vi "GetPackets.vi"(11 "ContextIn":T1={"COMHandler"="", "COMConfig"={"BaudRate"=9600, "DataBits"=8, "Parity"=enum."None", "StopBits"=10, "DataTransferTimeout[ms]"=10000, "FastTransferTimeout[ms]"=100, "Retries"=0, "MsWaitBeforeRetry"=0}, "HelloResponse"="", "DeviceDetected"=FALSE, "TransferRefusedByUser"=FALSE, "MeasurementFrequency"=0, "AvailablePacketsNr"=0, "RequestType"=enum."NONE", "Response"="", "DownloadSuccess"=FALSE, "PacketNames"=[], "Packets"=[], "ActivePacketID"=0} {"COMConfig"."StopBits" items=["1.0"=10, "1.5"=15, "2.0"=20]; "COMConfig"."DataBits" min=7 max=9 step=1; "COMConfig"."BaudRate" min=9600 max=921600 step=1}) -> (3 "ContextOut":T1={"COMHandler"="", "COMConfig"={"BaudRate"=9600, "DataBits"=8, "Parity"=enum."None", "StopBits"=10, "DataTransferTimeout[ms]"=10000, "FastTransferTimeout[ms]"=100, "Retries"=0, "MsWaitBeforeRetry"=0}, "HelloResponse"="", "DeviceDetected"=FALSE, "TransferRefusedByUser"=FALSE, "MeasurementFrequency"=0, "AvailablePacketsNr"=0, "RequestType"=enum."NONE", "Response"="", "DownloadSuccess"=FALSE, "PacketNames"=[], "Packets"=[], "ActivePacketID"=0} {"COMConfig"."StopBits" items=["1.0"=10, "1.5"=15, "2.0"=20]; "COMConfig"."DataBits" min=7 max=9 step=1; "COMConfig"."BaudRate" min=9600 max=921600 step=1})   [LabVIEW 2016]
doc: "Get all available packets. Packet by packet, decoding data frame on the fly."
uses:
  FSContext.ctl
  FTDI/COMConfig.ctl
  Requests/RequestType.ctl
  Packet.ctl
  Sample.ctl
  Reading.ctl
  ReadingUnits/AccelReadingUnit.ctl
  ReadingUnits/GyroReadingUnit.ctl
  GetPackets/GPState.ctl
  GetPackets/GPContext.ctl
panel:
  out "seconds remaining":u32
  out "Prompt":string
  in  "Download failed!":bool
  out "DownloadStatus":u8(slide) scale=0.0..99.0
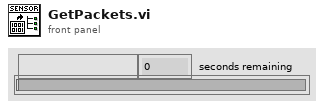
[diagram p1: front panel]
types:
  T1 = typedef "FSContext.ctl" = cluster{"COMHandler":refnum<visa-resource-name>, "COMConfig":T2, "HelloResponse":string, "DeviceDetected":bool, "TransferRefusedByUser":bool, "MeasurementFrequency":u32, "AvailablePacketsNr":u32, "RequestType":T3, "Response":string, "DownloadSuccess":bool, "PacketNames":string[], "Packets":T4[], "ActivePacketID":i32}
  T2 = typedef "COMConfig.ctl" = cluster{"BaudRate":u32, "DataBits":u16, "Parity":enum16{"None", "Odd", "Even", "Mark", "Space"}, "StopBits":u16, "DataTransferTimeout[ms]":u32, "FastTransferTimeout[ms]":u32, "Retries":i32, "MsWaitBeforeRetry":u32}
  T3 = typedef "RequestType.ctl" = enum16{"NONE", "Reset", "Hello", "GetPacketsNr", "GetMeasFreq", "GetPacket", "Goodbye"}
  T4 = typedef "Packet.ctl" = cluster{"Name":string, "SamplesNr":u32, "Samples":T5[], "AccelReadingUnit":T7, "GyroReadingUnit":T8}
  T5 = typedef "Sample.ctl" = cluster{"Accel":T6, "Gyro":T6}
  T6 = typedef "Reading.ctl" = cluster{"X":dbl, "Y":dbl, "Z":dbl}
  T7 = typedef "AccelReadingUnit.ctl" = enum16{"INVALID", "RAW", "g"}
  T8 = typedef "GyroReadingUnit.ctl" = enum16{"INVALID", "RAW", "°/sec"}
  T9 = typedef "GPContext.ctl" = cluster{"PacketsDownloaded":u32, "Millisecond":u32, "PacketsAfterNextSecond":u32}
  T10 = typedef "GPState.ctl" = enum16{"IDLE", "HandleErrors", "Init", "GetPacket", "UpdateDownloadSpeed", "UpdateProgress", "Stop"}
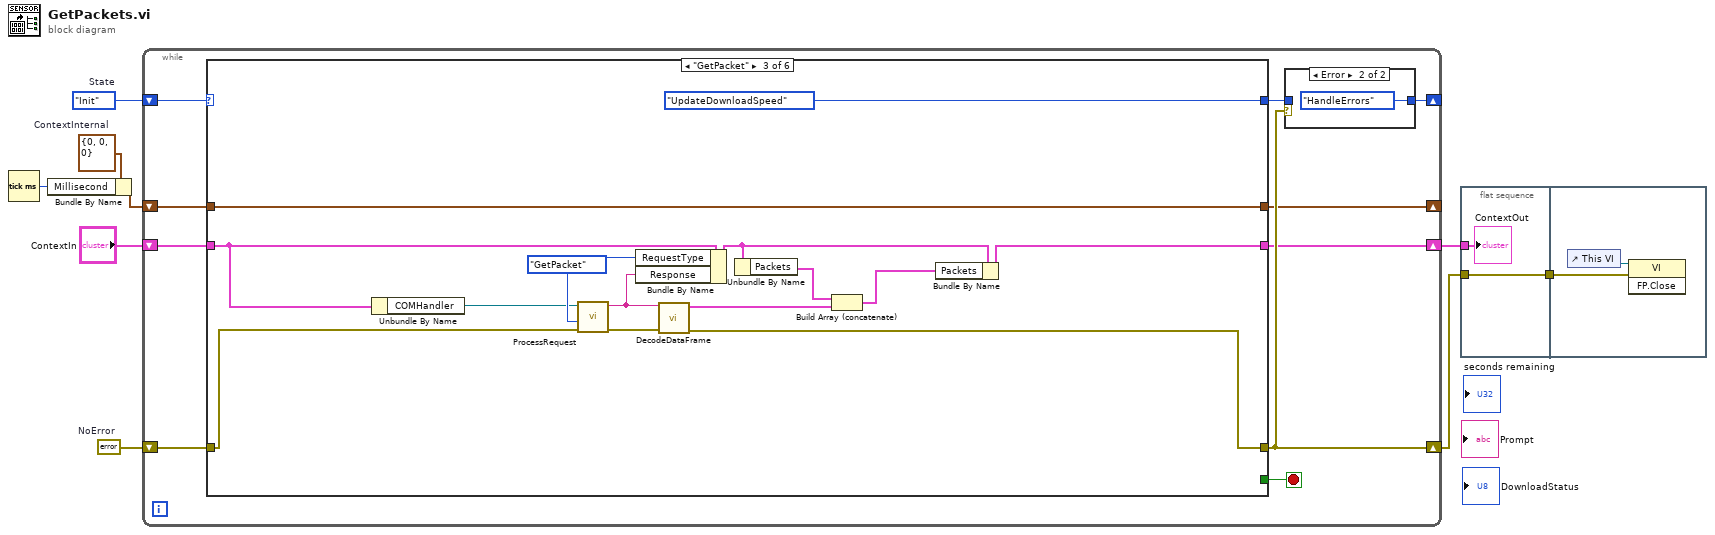
[diagram p0: block diagram]
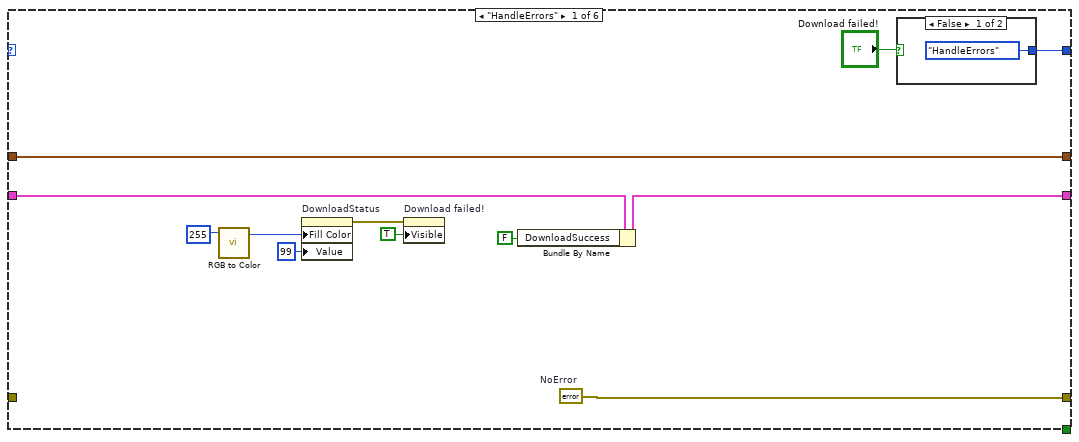
[diagram p3: hidden frame]
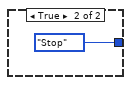
[diagram p4: hidden frame]
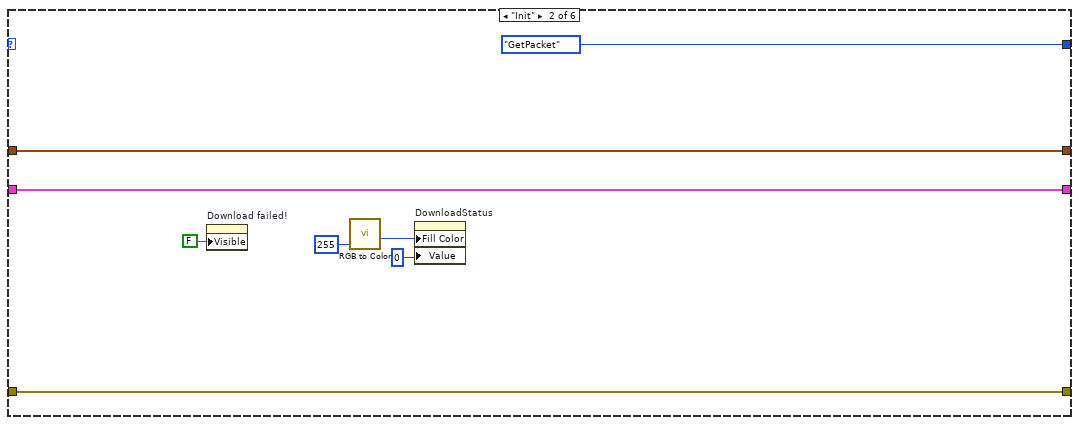
[diagram p5: hidden frame]
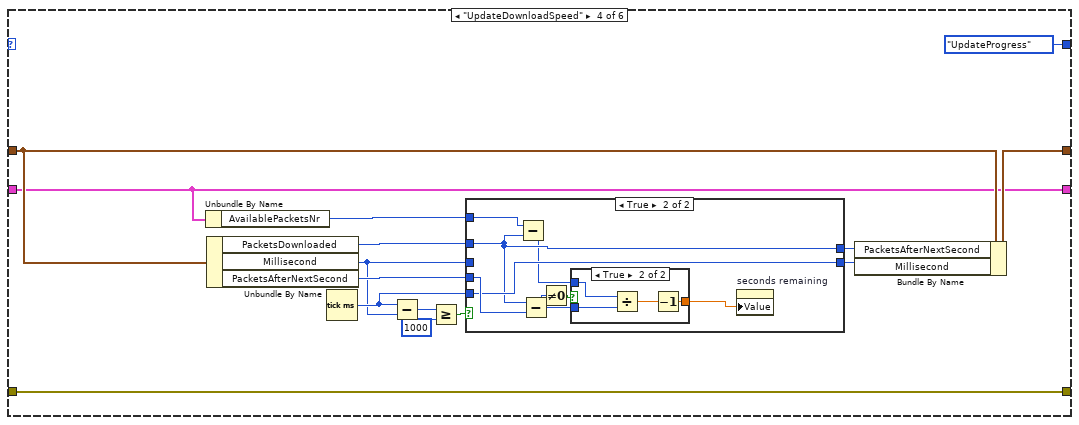
[diagram p6: hidden frame]
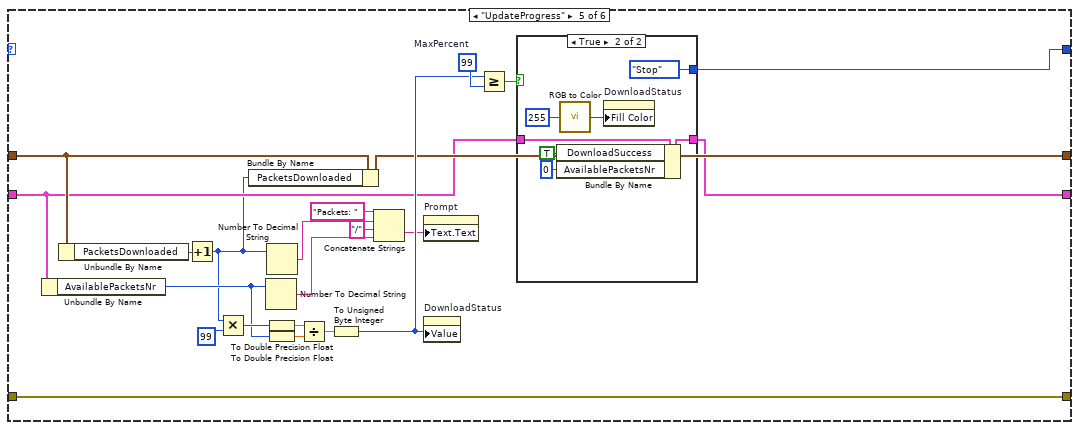
[diagram p9: hidden frame]
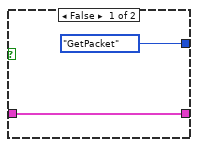
[diagram p10: hidden frame]
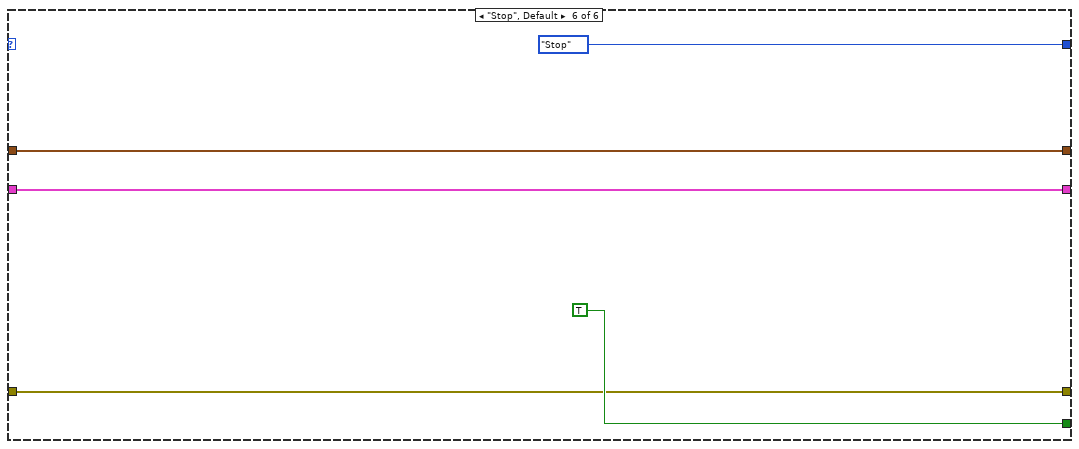
[diagram p11: hidden frame]
diagram:
  w4 = T9 {"PacketsDownloaded"=0, "Millisecond"=0, "PacketsAfterNextSecond"=0}  # ContextInternal
  w8 = errorcluster {"status"=FALSE, "code"=0, "source"=""}  # NoError
  w1 = GPState."Init"  # State
  n1 = Tick Count (ms)() -> (millisecond timer value=w3:u32)
  n2 = Bundle By Name(cluster=w4, "Millisecond"=w3) -> (w2:T9)
  n3 = while {
    shift-right: [w10] -> _
    shift-left: w1 -> [w11]
    shift-right: [w12] -> w7
    shift-left: "ContextIn" -> [w19]
    shift-right: [w15] -> w6
    shift-left: w8 -> [w18]
    shift-right: [w13] -> _
    shift-left: w2 -> [w14]
    stop <- w16 stop-if-true
    n4 = case shown="\"GetPacket\"" w11 {
      tunnel: w19 -> [w23 w41 w54 w59 w89 w120]
      tunnel: w18 -> [_ w43 w55 w62 w99 w121]
      tunnel: [w25 w43 w44 w62 w99 w121] -> w15
      tunnel: [w33 GPState."GetPacket" ("State") GPState."UpdateDownloadSpeed" ("State") GPState."UpdateProgress" ("State") w100 GPState."Stop" ("State")] -> w17
      tunnel: [_ _ _ _ _ TRUE] -> w16
      tunnel: [w22 w41 w45 w59 w88 w120] -> w12
      tunnel: w14 -> [w32 w36 w52 w65 w91 w118]
      tunnel: [w32 w36 w52 w64 w90 w118] -> w13
      frame "HandleErrors" {
        w25 = errorcluster {"status"=FALSE, "code"=0, "source"=""}  # NoError
        n5 = call <vilib>:"RGB to Color.vi"("R"=u8 255 ("G")) -> ("Color"=w30:u32)  [unwired: 2 in]
        n6 = property on="DownloadStatus" class="Slide (strict)"("Fill Color"=w30, "Value"=u8 99 ("DownloadStatus")) -> (error out=w29:errorcluster)  [unwired: 2 in, 1 out]
        n7 = property on="Download failed!" class="Bool"(error in=w29, "Visible"=TRUE) -> ()  [unwired: 1 in, 2 out]
        n8 = Bundle By Name(cluster=w23, "DownloadSuccess"=FALSE) -> (w22:T1)
        n9 = case shown="False" "Download failed!" {
          tunnel: [GPState."HandleErrors" ("State") GPState."Stop" ("State")] -> w33
          frame False {
          }
          frame True {
          }
        }
      }
      frame "Init" {
        n10 = property on="Download failed!" class="Bool"("Visible"=FALSE) -> ()  [unwired: 2 in, 2 out]
        n11 = call <vilib>:"RGB to Color.vi"("B"=u8 255 ("G")) -> ("Color"=w39:u32)  [unwired: 2 in]
        n12 = property on="DownloadStatus" class="Slide (strict)"("Fill Color"=w39, "Value"=u8 0 ("DownloadStatus")) -> ()  [unwired: 2 in, 2 out]
      }
      frame "GetPacket" {
        w57 = RequestType."GetPacket" ("RequestType")
        n13 = Unbundle By Name(w54) -> ("COMHandler"=w56:refnum<visa-resource-name>)
        n14 = call "ProcessRequest.vi"("ErrorIn"=w55, "RequestType"=w57, "DeviceResourceName"=w56) -> ("ErrorOut"=w50:errorcluster, "Response"=w51:string)  [unwired: 5 in, 2 out]
        n15 = Bundle By Name(cluster=w54, "RequestType"=w57, "Response"=w51) -> (w46:T1)
        n16 = call "DecodeDataFrame.vi"("ErrorIn"=w50, "Frame"=w51) -> ("ErrorOut"=w44:errorcluster, "Packets"=w49:T4[])  [unwired: 8 in]
        n17 = Unbundle By Name(w46) -> ("Packets"=w48:T4[])
        n18 = Build Array (concatenate)(w48, w49) -> (w47:T4[])
        n19 = Bundle By Name(cluster=w46, "Packets"=w47) -> (w45:T1)
      }
      frame "UpdateDownloadSpeed" {
        n20 = Unbundle By Name(w59) -> ("AvailablePacketsNr"=w58:u32)
        n21 = Unbundle By Name(w65) -> ("PacketsDownloaded"=w68:u32, "Millisecond"=w60:u32, "PacketsAfterNextSecond"=w69:u32)
        n22 = Tick Count (ms)() -> (millisecond timer value=w61:u32)
        n23 = Subtract(x=w61, y=w60) -> (x-y=w72:u32)
        n24 = Greater Or Equal?(x=w72, y=u32 1000) -> (x >= y?=w70:bool)
        n25 = case shown="True" w70 {
          tunnel: w69 -> [w73 w82]
          tunnel: w68 -> [_ w79]
          tunnel: [w73 w79] -> w67
          tunnel: w60 -> [w74 _]
          tunnel: [w74 w81] -> w66
          tunnel: w61 -> [_ w81]
          tunnel: w58 -> [_ w80]
          frame False {
          }
          frame True {
            n26 = Subtract(x=w80, y=w79) -> (x-y=w76:u32)
            n27 = Subtract(x=w79, y=w82) -> (x-y=w77:u32)
            n28 = Not Equal To 0?(x=w77) -> (x != 0?=w78:bool)
            n29 = case shown="True" w78 {
              tunnel: w77 -> [_ w85]
              tunnel: w76 -> [_ w86]
              tunnel: [_ w83] -> w75
              frame False {
              }
              frame True {
                n30 = Divide(x=w86, y=w85) -> (x/y=w84:dbl)
                n31 = Decrement(x=w84) -> (x-1=w83:dbl)
              }
            }
            n32 = property on="seconds remaining" class="DigNum (strict)"("Value"=w75) -> ()  [unwired: 2 in, 2 out]
          }
        }
        n33 = Bundle By Name(cluster=w65, "PacketsAfterNextSecond"=w67, "Millisecond"=w66) -> (w64:T9)
      }
      frame "UpdateProgress" {
        w103 = u8 99  # MaxPercent
        n34 = Unbundle By Name(w89) -> ("AvailablePacketsNr"=w93:u32)
        n35 = Unbundle By Name(w91) -> ("PacketsDownloaded"=w92:u32)
        n36 = Increment(x=w92) -> (x+1=w87:u32)
        n37 = Multiply(x=w87, y=u32 99) -> (x*y=w107:u32)
        n38 = Bundle By Name(cluster=w91, "PacketsDownloaded"=w87) -> (w90:T9)
        n39 = Number To Decimal String(number=w93) -> (decimal integer string=w97:string)  [unwired: 1 in]
        n40 = Number To Decimal String(number=w87) -> (decimal integer string=w96:string)  [unwired: 1 in]
        n41 = To Double Precision Float(number=w107) -> (double precision float=w106:dbl)
        n42 = To Double Precision Float(number=w93) -> (double precision float=w105:dbl)
        n43 = Divide(x=w106, y=w105) -> (x/y=w104:dbl)
        n44 = To Unsigned Byte Integer(number=w104) -> (unsigned 8bit integer=w102:u8)
        n45 = Concatenate Strings("Packets: " ("string"), w96, "/" ("string"), w97) -> (w98:string)
        n46 = property on="Prompt" class="Str"("Text.Text"=w98) -> ()  [unwired: 2 in, 2 out]
        n47 = property on="DownloadStatus" class="Slide (strict)"("Value"=w102) -> ()  [unwired: 2 in, 2 out]
        n48 = Greater Or Equal?(x=w102, y=w103) -> (x >= y?=w101:bool)
        n49 = case shown="True" w101 {
          tunnel: [GPState."GetPacket" ("State") GPState."Stop" ("State")] -> w100
          tunnel: w89 -> [w109 w113]
          tunnel: [w109 w112] -> w88
          frame False {
          }
          frame True {
            n50 = Bundle By Name(cluster=w113, "DownloadSuccess"=TRUE, "AvailablePacketsNr"=u32 0) -> (w112:T1)
            n51 = call <vilib>:"RGB to Color.vi"("G"=u8 255) -> ("Color"=w115:u32)  [unwired: 2 in]
            n52 = property on="DownloadStatus" class="Slide (strict)"("Fill Color"=w115) -> ()  [unwired: 2 in, 2 out]
          }
        }
      }
      frame "Stop", Default {
      }
    }
    n53 = case shown="Error" w15 {
      tunnel: w17 -> [w20 _]
      tunnel: [w20 GPState."HandleErrors" ("State")] -> w10
      frame No Error {
      }
      frame Error {
      }
    }
  }
  n54 = flat-sequence {
    tunnel: w7 -> [w124]
    tunnel: w6 -> [w123]
    tunnel: [w123] -> w5
    tunnel: w5 -> [w125]
    frame #0 {
      "ContextOut" <- w124
    }
    frame #1 {
      n55 = control-ref of="This VI"() -> (w126:refnum<vi>)
      n56 = invoke class="VI" method="FP.Close"(reference=w126, error in=w125) -> ()  [unwired: 1 in, 3 out]
    }
  }
